vi "Com_Matrix220_Read Message.vi"(8 "error in":errorcluster, 11 "Buffer Data In":T2) -> (0 "error out":errorcluster, 1 "Timeout?":bool, 2 "Message":string, 3 "Buffer Data Out":T2, 4 "Message Type":T1=enum."Code")   [LabVIEW 2016]
uses:
  Data Def/Com_Matrix220_Buffer Data.ctl
  Data Def/Com_Matrix220_Message Type.ctl
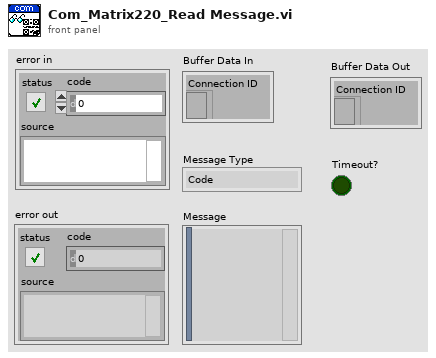
[diagram p1: front panel]
types:
  T1 = typedef "Com_Matrix220_Message Type.ctl" = enum16{"Unkown", "Ack", "Code", "Image"}
  T2 = typedef "Com_Matrix220_Buffer Data.ctl" = cluster{"Connection ID":refnum<k5>}
  T3 = enum16{"Standard", "Buffered", "CRLF", "Immediate"}
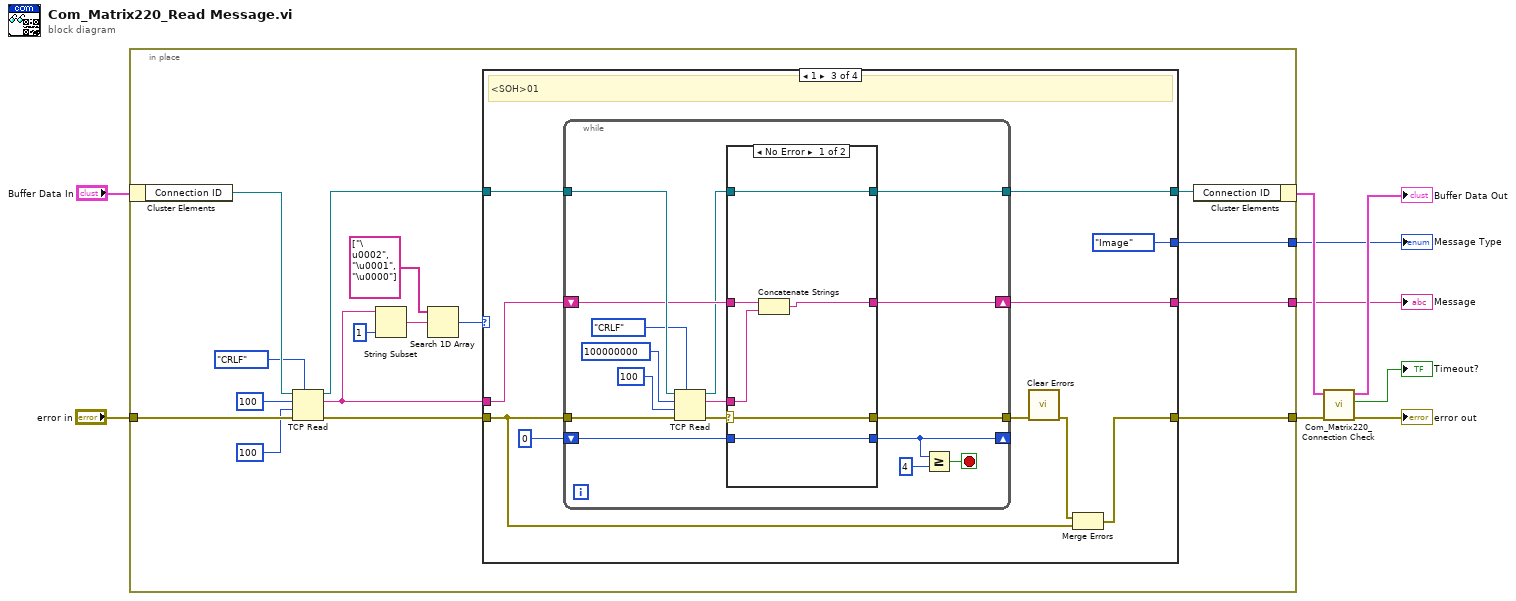
[diagram p0: block diagram]
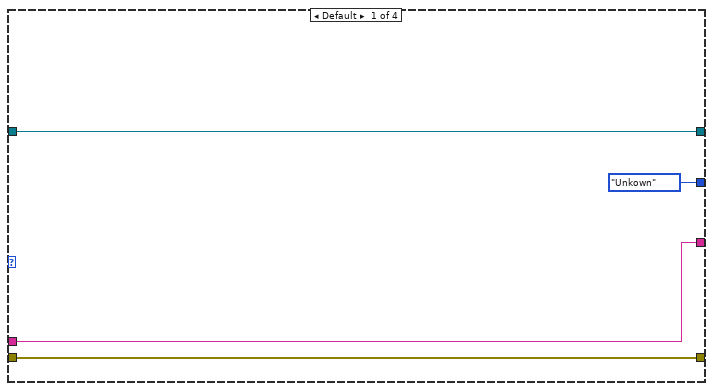
[diagram p2: hidden frame]
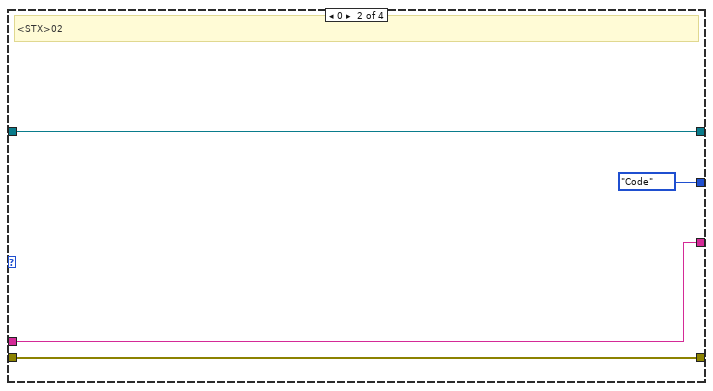
[diagram p3: hidden frame]
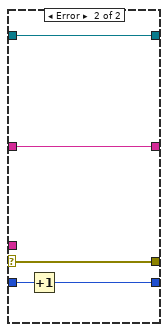
[diagram p4: hidden frame]
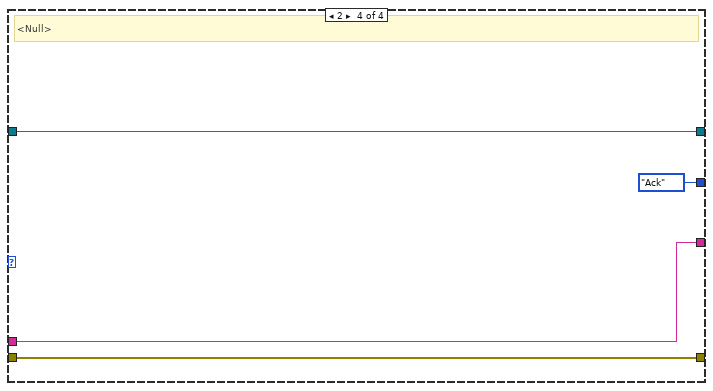
[diagram p5: hidden frame]
diagram:
  n1 = in-place {
    in-place-border: "error in" -> [w23]
    in-place-border: [w15] -> w7
    in-place-border: [w13] -> w2
    in-place-border: [w12] -> w1
    n2 = in-place-cluster #1("Buffer Data In") -> ("Connection ID"=w25:refnum<k5>)
    n3 = TCP Read(connection ID=w25, bytes to read=100, error in (no error)=w23, 7:T3."CRLF" ("mode (standard)"), 9:100 ("timeout ms (25000)")) -> (connection ID out=w11:refnum<k5>, data out=w14:string, error out=w17:errorcluster)
    n4 = String Subset(string=w14, length (rest)=1 ("length (rest)")) -> (substring=w19:string)  [unwired: 1 in]
    n5 = Search 1D Array(1D array=string[] ["\u0002", "\u0001", "\u0000"], element=w19) -> (index of element=w16:i32)  [unwired: 1 in]
    n6 = case shown="1" w16 {
      tunnel: w17 -> [w29 w33 w35 w73]
      tunnel: [w29 w33 w34 w73] -> w15
      tunnel: w14 -> [w27 w30 w41 w71]
      tunnel: [w27 w30 w37 w71] -> w13
      tunnel: [Com_Matrix220_Message_Type."Unkown" ("Message Type") Com_Matrix220_Message_Type."Code" ("Message Type") Com_Matrix220_Message_Type."Image" ("Message Type") Com_Matrix220_Message_Type."Ack" ("Message Type")] -> w12
      tunnel: w11 -> [w26 w31 w42 w72]
      tunnel: [w26 w31 w40 w72] -> w10
      frame Default {
      }
      frame 0 {
        # "<STX>02"
      }
      frame 1 {
        # "<SOH>01"
        n7 = while {
          tunnel: w35 -> [w59]
          tunnel: w42 -> [w56]
          shift-right: [w49] -> w37
          shift-left: w41 -> [w54]
          tunnel: [w50] -> w40
          shift-right: [w47] -> _
          shift-left: 0 -> [w48]
          tunnel: [w44] -> w38
          stop <- w45 stop-if-true
          n8 = TCP Read(connection ID=w56, bytes to read=100000000, error in (no error)=w59, 7:T3."CRLF" ("mode (standard)"), 9:100 ("timeout ms (25000)")) -> (connection ID out=w51:refnum<k5>, data out=w52:string, error out=w55:errorcluster)
          n9 = case shown="No Error" w55 {
            selector: w55 -> [w61 w68]
            tunnel: w54 -> [w64 w70]
            tunnel: w52 -> [w63 _]
            tunnel: w51 -> [w65 w69]
            tunnel: [w65 w69] -> w50
            tunnel: [w62 w70] -> w49
            tunnel: [w61 w68] -> w44
            tunnel: w48 -> [w60 w67]
            tunnel: [w60 w66] -> w47
            frame No Error {
              n10 = Concatenate Strings(w64, w63) -> (w62:string)
            }
            frame Error {
              n11 = Increment(x=w67) -> (x+1=w66:i32)
            }
          }
          n12 = Greater Or Equal?(x=w47, y=4) -> (x >= y?=w45:bool)
        }
        n13 = call <vilib>:"Clear Errors.vi"("error in (no error)"=w38) -> ("error out"=w36:errorcluster)  [unwired: 5 in, 1 out]
        n14 = Merge Errors(w36, w35) -> (w34:errorcluster)
      }
      frame 2 {
        # "<Null>"
      }
    }
    n15 = in-place-cluster #1("Connection ID"=w10) -> (w6:T2)
  }
  "Message" <- w2
  "Message Type" <- w1
  n16 = call "Com_Matrix220_Connection Check.vi"("error in"=w7, "Buffer Data In"=w6) -> ("error out"=→"error out":errorcluster, "Timeout?"=→"Timeout?":bool, "Buffer Data Out"=→"Buffer Data Out":T2)  [unwired: 7 in]
